vi "总磷氨氮插入数据.vi"(0 "table":string, 5 "data":T2={"时间标识"=timestamp(0 s since 1904-01-01), "测量模式"=enum."水样测试", "数据标记表"="N", "监测值"=0.0, "单位"=0, "数据标识"="", "因子编码"=0, "标样参考值"=0.0, "F0"=0.0, "F1"=0.0, "F2"=0.0, "F3"=0.0, "F4"=0.0, "F5"=0.0, "F6"=0.0, "F7"=0.0, "X"=0.0, "温度"=0.0, "湿度"=0.0, "量程标识"="", "SN"="", "跨度值"=0.0} {"单位" items=["μg/L", "mg/L", "ppm", "mg/m3", "cm", "ppb", "μg/m3", "%", "nmol/mol", "μmol/mol", "MPN/L", "MPN/100ml", "ng/m3", "NTU", "无量纲", "ms/cm", "μs/cm"]}, 11 "error in (no error)":errorcluster) -> (15 "error out":errorcluster)   [LabVIEW 2016, in "斯坦道总磷.lvlib"]
uses:
  <vilib>/Utility/sysdir.llb/System Directory Type.ctl
  <vilib>/Utility/error.llb/DialogType.ctl
  <vilib>/addons/database/Auxilliary.llb/DB Tools Column Info.ctl
  <vilib>/addons/database/Auxilliary.llb/DB Tools DataTypes.ctl
  <vilib>/addons/database/Connection.llb/DB Tools Open Connec (String).vi
  <vilib>/addons/database/Connection.llb/Conn Execute.vi
  <vilib>/addons/database/Recordset.llb/Rec Fetch Recordset Data (R).vi
  <vilib>/addons/database/Recordset.llb/Rec Destroy - Connection.vi
  <vilib>/addons/database/NI_Database_API.lvlib
panel:
  out "data输出":T1
  out "为空？":bool
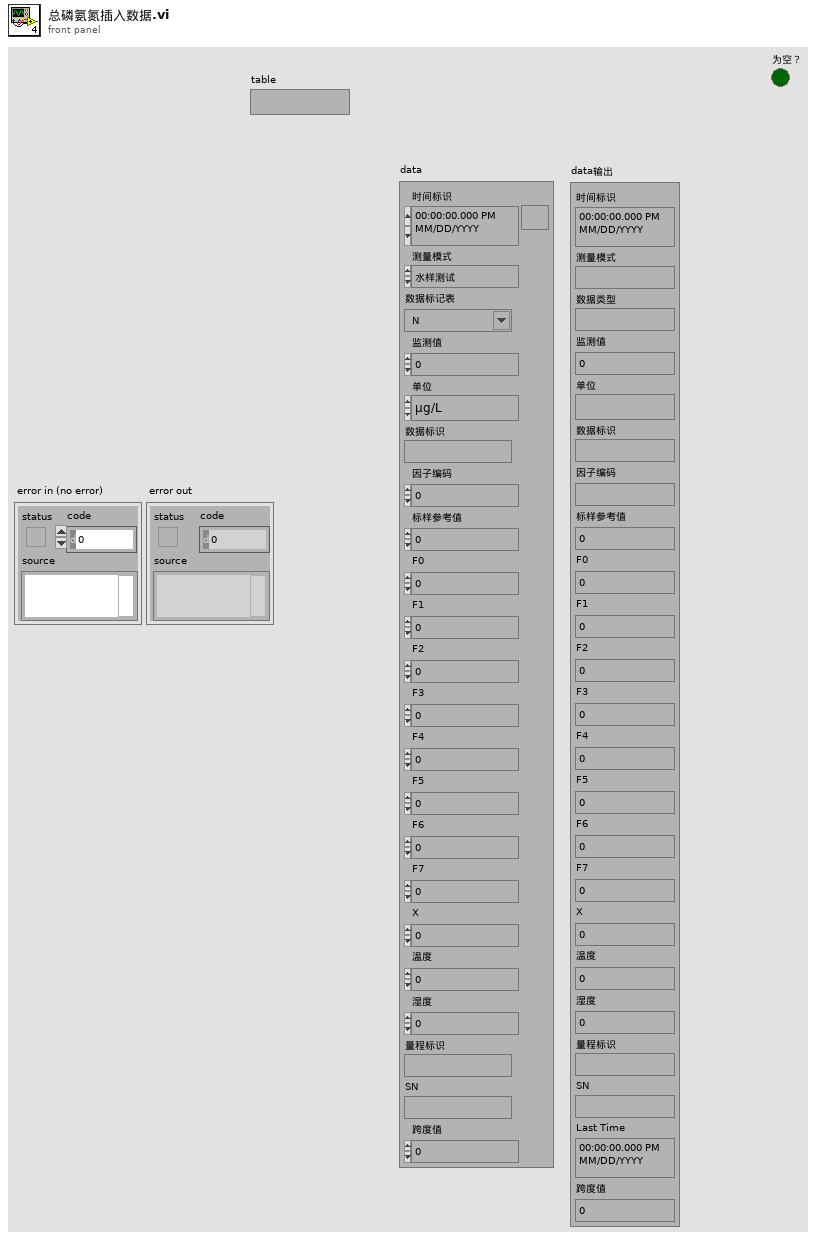
[diagram p1: front panel]
types:
  T1 = cluster{"时间标识":timestamp, "测量模式":string, "数据类型":string, "监测值":sgl, "单位":string, "数据标识":string, "因子编码":string, "标样参考值":sgl, "F0":sgl, "F1":sgl, "F2":sgl, "F3":sgl, "F4":sgl, "F5":sgl, "F6":sgl, "F7":sgl, "X":sgl, "温度":sgl, "湿度":sgl, "量程标识":string, "SN":string, "Last Time":timestamp, "跨度值":sgl}
  T2 = cluster{"时间标识":timestamp, "测量模式":enum16{"维护数据", "水样测试", "标样核查", "零点核查", "跨度核查", "空白测试", "平行样测试", "加标回收", "空白校准", "标样校准", "初始化（清洗）"}, "数据标记表":string, "监测值":sgl, "单位":u16, "数据标识":string, "因子编码":u32, "标样参考值":sgl, "F0":sgl, "F1":sgl, "F2":sgl, "F3":sgl, "F4":sgl, "F5":sgl, "F6":sgl, "F7":sgl, "X":sgl, "温度":sgl, "湿度":sgl, "量程标识":string, "SN":string, "跨度值":sgl}
  T3 = typedef "DialogType.ctl" = u16
  T4 = typedef "System Directory Type.ctl" = i32
  T5 = typedef "NI_Database_API.lvlib/Conn ObjectReference.ctl" = refnum<k1>
  T6 = typedef "NI_Database_API.lvlib/Rec ObjectReference.ctl" = refnum<k1>
  T7 = typedef "NI_Database_API.lvlib/DB Tools Column Info.ctl" = cluster{"column name":string, "data type":T8, "size":i32, "allow null?":bool}
  T8 = typedef "NI_Database_API.lvlib/DB Tools DataTypes.ctl" = enum16{"String", "Long (I32)", "Single (SGL)", "Double (DBL)", "Date/Time", "Binary"}
  T9 = enum16{"维护数据", "水样测试", "标样核查", "零点核查", "跨度核查", "空白测试", "平行样测试", "加标回收", "空白校准", "标样校准", "初始化（清洗）"}
  T10 = cluster{"测量量程":dbl, "测量精度":dbl, "测量间隔":dbl, "消解温度":dbl, "消解时长":dbl, "空白校准时间":timestamp, "曲线截距":dbl, "曲线斜率":dbl, "测量检出限":dbl, "测量信号值":dbl, "线性相关系数":dbl, "二次多项式系数":dbl, "标样校准时间":timestamp, "稀释倍数":dbl, "三项式系数":dbl, "空白标定系数":dbl, "量程系数":dbl, "F0/ORPA":dbl, "F1/ORPB":dbl, "F2/ORPK":dbl, "F3":dbl, "F4":dbl, "F5":dbl, "F6":dbl, "F7":dbl, "X0/滴定数":dbl, "量程":dbl}
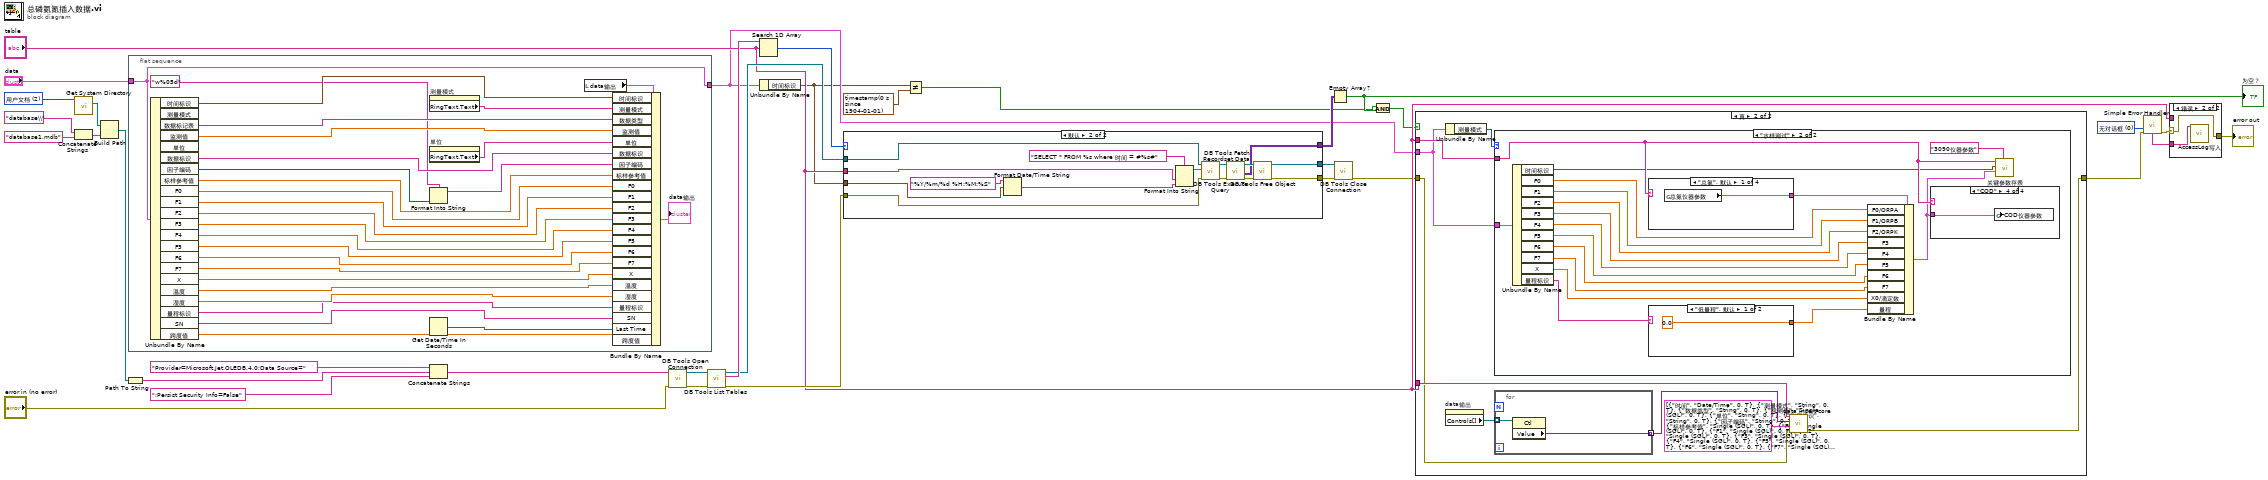
[diagram p0: block diagram]
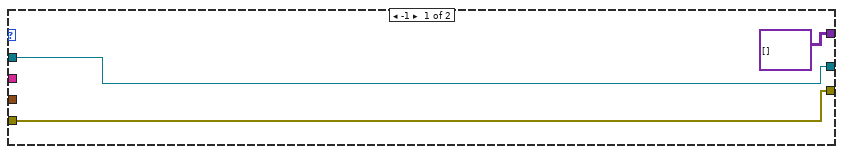
[diagram p3: hidden frame]
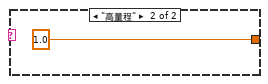
[diagram p6: hidden frame]
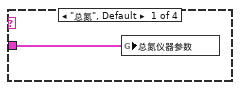
[diagram p7: hidden frame]
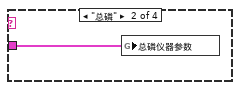
[diagram p8: hidden frame]
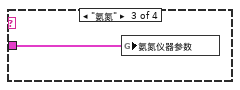
[diagram p9: hidden frame]
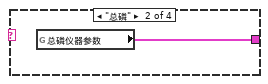
[diagram p10: hidden frame]
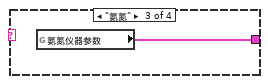
[diagram p11: hidden frame]
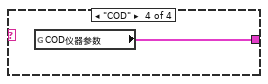
[diagram p12: hidden frame]
diagram:
  w15 = T3 0 items=["无对话框", "确定信息", "继续或停止信息", "确定信息＋警告", "继续/停止+警告"] ("type of dialog (OK msg:1)")
  w33 = T4 2 items=["用户目录"=0, "用户桌面"=1, "用户文档"=2, "用户应用程序数据"=3, "用户设置"=4, "用户临时目录"=5, "公共文档"=6, "公共应用程序数据"=7, "公共设置"=8, "公共缓存"=13, "系统核心库"=9, "系统安装库"=10, "应用程序文件"=11, "启动盘根目录"=12] ("system directory type")
  n1 = call <vilib>:"Get System Directory.vi"("system directory type"=w33) -> ("system directory"=w31:path)  [unwired: 10 in]
  n2 = Concatenate Strings("database\\" ("condition"), "database1.mdb" ("database")) -> (w25:string)
  n3 = Build Path(base path=w31, name or relative path=w25) -> (appended path=w30:path)
  n4 = Path To String(path=w30) -> (string=w29:string)
  n5 = flat-sequence {
    tunnel: "data" -> [w40]
    tunnel: [w40] -> w9
    frame #0 {
      n6 = Unbundle By Name(w40) -> ("时间标识"=w61:timestamp, "数据标记表"=w59:string, "监测值"=w58:sgl, "数据标识"=w56:string, "因子编码"=w39:u32, "标样参考值"=w55:sgl, "F0"=w54:sgl, "F1"=w53:sgl, "F2"=w52:sgl, "F3"=w51:sgl, "F4"=w50:sgl, "F5"=w49:sgl, "F6"=w48:sgl, "F7"=w47:sgl, "X"=w46:sgl, "温度"=w45:sgl, "湿度"=w44:sgl, "量程标识"=w43:string, "SN"=w42:string, "跨度值"=w35:sgl)  [unwired: 2 out]
      n7 = property on="测量模式" class="Enum (严格)"() -> ("RingText.Text"=w60:string)  [unwired: 2 in, 2 out]
      n8 = property on="单位" class="Ring (严格)"() -> ("RingText.Text"=w57:string)  [unwired: 2 in, 2 out]
      n9 = Format Into String(format string="w%05d" ("格式字符串"), w39) -> (resulting string=w37:string)  [unwired: 2 in, 1 out]
      n10 = Get Date/Time In Seconds() -> (seconds since 1Jan1904=w41:timestamp)
      n11 = local read "data输出"() -> (w36:T1)
      n12 = Bundle By Name(cluster=w36, "时间标识"=w61, "测量模式"=w60, "数据类型"=w59, "监测值"=w58, "单位"=w57, "数据标识"=w56, "因子编码"=w37, "标样参考值"=w55, "F0"=w54, "F1"=w53, "F2"=w52, "F3"=w51, "F4"=w50, "F5"=w49, "F6"=w48, "F7"=w47, "X"=w46, "温度"=w45, "湿度"=w44, "量程标识"=w43, "SN"=w42, "Last Time"=w41, "跨度值"=w35) -> (→"data输出":T1)
    }
  }
  n13 = Concatenate Strings("Provider=Microsoft.Jet.OLEDB.4.0;Data Source=" ("condition"), w29, ";Persist Security Info=False" ("condition")) -> (w27:string)
  n14 = call-poly <vilib>:"DB Tools Open Connection.vi"("error in (no error)"="error in (no error)", "connection information"=w27) -> ("error out"=w23:errorcluster, "connection reference"=w24:T5)  [unwired: 6 in]
  n15 = call <vilib>:"DB Tools List Tables.vi"("error in (no error)"=w23, "connection reference"=w24) -> ("error out"=w17:errorcluster, "tables"=w22:string[], "connection reference out"=w18:T5)  [unwired: 3 in]
  n16 = Search 1D Array(1D array=w22, element="table") -> (index of element=w19:i32)  [unwired: 1 in]
  n17 = Unbundle By Name(w9) -> ("时间标识"=w7:timestamp)
  n18 = case shown="默认" w19 {
    tunnel: [variant[][] [] ("recordset data") w76] -> w16
    tunnel: [w65 w67] -> w4
    tunnel: [w64 w75] -> w3
    tunnel: w18 -> [w65 w71]
    tunnel: w17 -> [w64 w70]
    tunnel: "table" -> [_ w69]
    tunnel: w7 -> [_ w66]
    frame -1 {
    }
    frame Default {
      n19 = Format Date/Time String(time format string (%c)="%Y/%m/%d %H:%M:%S" ("时间格式字符串(%c)"), seconds (now)=w66) -> (date/time string=w72:string)  [unwired: 1 in]
      n20 = Format Into String(format string="SELECT * FROM %s where 时间 = #%s#" ("格式字符串"), w69, w72) -> (resulting string=w74:string)  [unwired: 2 in, 1 out]
      n21 = call-poly <vilib>:"DB Tools Execute Query.vi"("error in (no error)"=w70, "SQL query"=w74, "connection reference"=w71) -> ("error out"=w77:errorcluster, "recordset reference"=w80:T6)  [unwired: 5 in]
      n22 = call-poly <vilib>:"DB Tools Fetch Recordset Data.vi"("error in (no error)"=w77, "recordset reference"=w80) -> ("error out"=w78:errorcluster, "recordset data"=w76:variant[][], "recordset reference out"=w79:T6)  [unwired: 3 in]
      n23 = call-poly <vilib>:"DB Tools Free Object.vi"("error in (no error)"=w78, "recordset reference"=w79) -> ("error out"=w75:errorcluster, "connection reference"=w67:T5)  [unwired: 8 in]
    }
  }
  n24 = Not Equal?(x=w7, y=timestamp(0 s since 1904-01-01)) -> (x != y?=w5:bool)
  n25 = Empty Array?(array=w16) -> (empty?=w20:bool)
  "为空？" <- w20
  n26 = call <vilib>:"DB Tools Close Connection.vi"("error in (no error)"=w3, "connection reference"=w4) -> ("error out"=w2:errorcluster)  [unwired: 5 in]
  n27 = And(x=w5, y=w20) -> (x .and. y?=w6:bool)
  n28 = case shown="真" w6 {
    tunnel: "table" -> [_ w86]
    tunnel: w9 -> [_ w83]
    tunnel: w2 -> [w81 w85]
    tunnel: [w81 w84] -> w1
    tunnel: "table" -> [_ w90]
    frame False {
    }
    frame True {
      n29 = Unbundle By Name(w83) -> ("测量模式"=w82:T9)
      n30 = property on="data输出" class="Clust (严格)"() -> ("Controls[]"=w87:refnum<vi>[])  [unwired: 2 in, 2 out]
      n31 = case shown="\"水样测试\"" w82 {
        tunnel: w83 -> [_ w108]
        tunnel: w90 -> [_ w106]
        frame "维护数据", Default {
        }
        frame "水样测试" {
          n32 = Unbundle By Name(w108) -> ("时间标识"=w104:timestamp, "F0"=w93:sgl, "F1"=w94:sgl, "F2"=w95:sgl, "F3"=w96:sgl, "F4"=w97:sgl, "F5"=w98:sgl, "F6"=w99:sgl, "F7"=w100:sgl, "X"=w101:sgl, "量程标识"=w103:string)
          n33 = case shown="\"总氮\", 默认" w106 {
            tunnel: [w116 w117 w118 w119] -> w107
            frame "总氮", Default {
              n34 = global read "总磷总氮断电保存全局变量.vi" "总氮仪器参数"() -> (w116:T10)
            }
            frame "总磷" {
              n35 = global read "总磷总氮断电保存全局变量.vi" "总磷仪器参数"() -> (w117:T10)
            }
            frame "氨氮" {
              n36 = global read "总磷总氮断电保存全局变量.vi" "氨氮仪器参数"() -> (w118:T10)
            }
            frame "COD" {
              n37 = global read "总磷总氮断电保存全局变量.vi" "COD仪器参数"() -> (w119:T10)
            }
          }
          n38 = case shown="\"低量程\", 默认" w103 {
            tunnel: [0.0 1.0] -> w102
            frame "低量程", Default {
            }
            frame "高量程" {
            }
          }
          n39 = Bundle By Name(cluster=w107, "F0/ORPA"=w93, "F1/ORPB"=w94, "F2/ORPK"=w95, "F3"=w96, "F4"=w97, "F5"=w98, "F6"=w99, "F7"=w100, "X0/滴定数"=w101, "量程"=w102) -> (w105:T10)
          n40 = case shown="\"COD\"" w106 {
            tunnel: w105 -> [w112 w113 w114 w115]
            frame "总氮", Default {
              n41 = global write "总磷总氮断电保存全局变量.vi" "总氮仪器参数"(w112) -> ()
            }
            frame "总磷" {
              n42 = global write "总磷总氮断电保存全局变量.vi" "总磷仪器参数"(w113) -> ()
            }
            frame "氨氮" {
              n43 = global write "总磷总氮断电保存全局变量.vi" "氨氮仪器参数"(w114) -> ()
            }
            frame "COD" {
              n44 = global write "总磷总氮断电保存全局变量.vi" "COD仪器参数"(w115) -> ()
            }
          }
          n45 = call "关键参数存表.vi"("table"="3090仪器参数", "仪器参数"=w105, "datatime"=w104, "仪器名称"=w106) -> ()  [unwired: 7 in, 1 out]
        }
      }
      n46 = for {
        tunnel: w87 -> [w92] mode=indexing
        tunnel: [w91] -> w89 mode=indexing
        n47 = property class="Ctl"(reference=w92) -> ("Value"=w91:variant)  [unwired: 1 in, 2 out]
      }
      n48 = call "data insert core.vi"("error in (no error)"=w85, "column information"=T7[] [{"column name"="时间", "data type"=enum."Date/Time", "size"=0, "allow null?"=TRUE}, {"column name"="测量模式", "data type"=enum."String", "size"=0, "allow null?"=TRUE}, {"column name"="数据类型", "data type"=enum."String", "size"=0, "allow null?"=TRUE}, {"column name"="检测值", "data type"=enum."Single (SGL)", "size"=0, "allow null?"=TRUE}, {"column name"="单位", "data type"=enum."String", "size"=0, "allow null?"=TRUE}, {"column name"="数据标识", "data type"=enum."String", "size"=0, "allow null?"=TRUE}, {"column name"="因子编码", "data type"=enum."String", "size"=0, "allow null?"=TRUE}, {"column name"="标样参考值", "data type"=enum."Single (SGL)", "size"=0, "allow null?"=TRUE}, {"column name"="F0", "data type"=enum."Single (SGL)", "size"=0, "allow null?"=TRUE}, {"column name"="F1", "data type"=enum."Single (SGL)", "size"=0, "allow null?"=TRUE}, {"column name"="F2", "data type"=enum."Single (SGL)", "size"=0, "allow null?"=TRUE}, {"column name"="F3", "data type"=enum."Single (SGL)", "size"=0, "allow null?"=TRUE}, {"column name"="F4", "data type"=enum."Single (SGL)", "size"=0, "allow null?"=TRUE}, {"column name"="F5", "data type"=enum."Single (SGL)", "size"=0, "allow null?"=TRUE}, {"column name"="F6", "data type"=enum."Single (SGL)", "size"=0, "allow null?"=TRUE}, {"column name"="F7", "data type"=enum."Single (SGL)", "size"=0, "allow null?"=TRUE}, {"column name"="X", "data type"=enum."Single (SGL)", "size"=0, "allow null?"=TRUE}, {"column name"="温度", "data type"=enum."Single (SGL)", "size"=0, "allow null?"=TRUE}, {"column name"="湿度", "data type"=enum."Single (SGL)", "size"=0, "allow null?"=TRUE}, {"column name"="量程标识", "data type"=enum."String", "size"=0, "allow null?"=TRUE}, {"column name"="SN", "data type"=enum."String", "size"=0, "allow null?"=TRUE}, {"column name"="LastTime", "data type"=enum."Date/Time", "size"=0, "allow null?"=TRUE}, {"column name"="跨度值", "data type"=enum."Single (SGL)", "size"=0, "allow null?"=TRUE}], "data"=w89, "table"=w86) -> ("error out"=w84:errorcluster)  [unwired: 7 in]
    }
  }
  n49 = call <vilib>:"Simple Error Handler.vi"("type of dialog (OK msg:1)"=w15, "error in (no error)"=w1) -> ("error out"=w14:errorcluster, "message"=w13:string)  [unwired: 3 in, 3 out]
  n50 = case shown="错误" w14 {
    selector: w14 -> [_ w120]
    tunnel: w13 -> [_ w121]
    tunnel: [_ w120] -> w12
    tunnel: "table" -> [_ _]
    frame No Error {
    }
    frame Error {
      n51 = call "AccessLog写入.vi"("Log"=w121) -> ()  [unwired: 11 in]
    }
  }
  "error out" <- w12
